vi "Read Internet INI.vi"(7 "section":string, 8 "error in (no error)":errorcluster, 10 "defaults":string[](array[string]), 11 "tokens":string[](array[string])) -> (0 "error out":errorcluster, 3 "values":string[](array[string]))   [LabVIEW 2017, in "NI_FTP.lvlib"]
uses:
  <vilib>/FTP/NI_FTP.lvlib
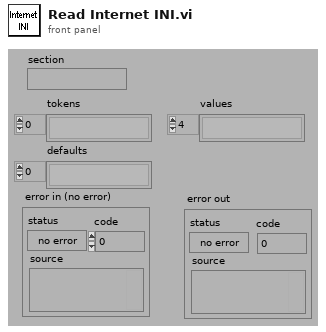
[diagram p1: front panel]
types:
  T1 = typedef "NI_FTP.lvlib/Keyed Array.ctl" = cluster{"keys":string[], "values":string[]}
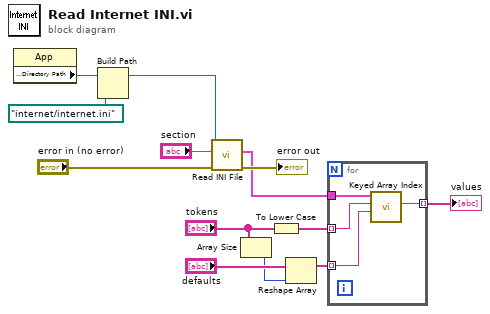
[diagram p0: block diagram]
diagram:
  n1 = property class="App"() -> ("Application:Directory Path"=w1:path)  [unwired: 2 in, 2 out]
  n2 = Build Path(base path=w1, name or relative path=path "internet/internet.ini") -> (appended path=w12:path)
  n3 = call <vilib>:"Read INI File.vi"("error in (no error)"="error in (no error)", "section"="section", "ini file path"=w12) -> ("error out"=→"error out":errorcluster, "keyed array"=w8:T1)  [unwired: 1 in, 6 out]
  n4 = Array Size(array="tokens") -> (size(s)=w3:i32)
  n5 = To Lower Case(string="tokens") -> (all lower case string=w2:string[])
  n6 = Reshape Array("defaults", w3) -> (w5:string[])
  n7 = for {
    tunnel: w8 -> [w17]
    tunnel: w2 -> [w16] mode=indexing
    tunnel: w5 -> [w15] mode=indexing
    tunnel: [w14] -> w7 mode=indexing
    n8 = call <vilib>:"Keyed Array Index.vi"("default value"=w15, "key"=w16, "array in"=w17) -> ("value"=w14:string)  [unwired: 1 in, 3 out]
  }
  "values" <- w7
